vi "Send Command.vi"(6 "bytes to read":i32=256, 8 "error in (no error)":errorcluster, 9 "Get responce":bool=TRUE, 10 "Command":string="Version", 11 "RFSoC Driver in":refnum<class "RFSoC Driver.lvclass">) -> (0 "error out":errorcluster, 2 "Responce":string, 3 "RFSoC Driver out":refnum<class "RFSoC Driver.lvclass">)   [LabVIEW 2019, in "RFSoC Driver.lvclass"]
uses:
  RFSoC Driver.lvclass
  RFSoC Driver.lvclass/RFSoC Driver.ctl
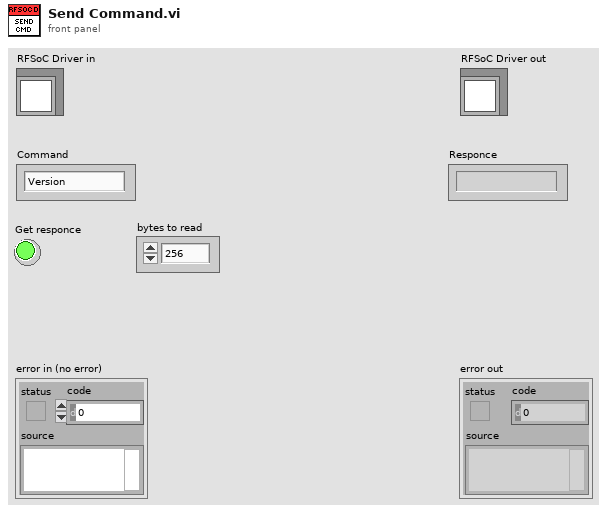
[diagram p1: front panel]
types:
  T1 = enum16{"Standard", "Buffered", "CRLF", "Immediate"}
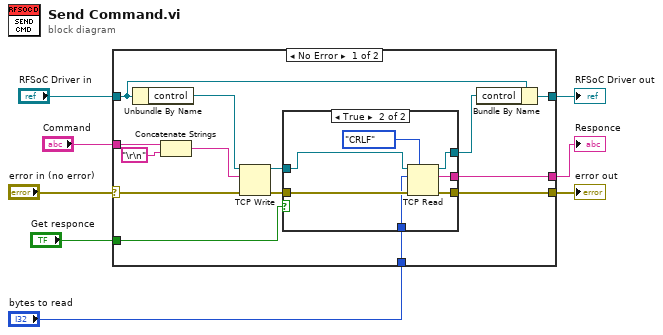
[diagram p0: block diagram]
diagram:
  n1 = case shown="No Error" "error in (no error)" {
    selector: "error in (no error)" -> [w17 w33]
    tunnel: [w14 w33] -> w7
    tunnel: [w12 w32] -> w5
    tunnel: "RFSoC Driver in" -> [w22 w32]
    tunnel: "Command" -> [w20 _]
    tunnel: "Get responce" -> [w16 _]
    tunnel: [w10 _] -> w2
    tunnel: "bytes to read" -> [w9 _]
    frame No Error {
      n2 = Unbundle By Name(w22) -> ("control"=w21:refnum<k5>)
      n3 = Concatenate Strings(w20, "\r\n") -> (w18:string)
      n4 = TCP Write(connection ID=w21, data in=w18, error in (no error)=w17) -> (connection ID out=w13:refnum<k5>, error out=w15:errorcluster)  [unwired: 1 in, 1 out]
      n5 = case shown="True" w16 {
        tunnel: w15 -> [w24 w30]
        tunnel: [w24 w29] -> w14
        tunnel: w13 -> [w23 w28]
        tunnel: [w23 w27] -> w11
        tunnel: [_ w26] -> w10
        tunnel: w9 -> [_ w25]
        frame False {
        }
        frame True {
          n6 = TCP Read(connection ID=w28, bytes to read=w25, error in (no error)=w30, 7:T1."CRLF" ("mode (standard)")) -> (connection ID out=w27:refnum<k5>, data out=w26:string, error out=w29:errorcluster)  [unwired: 1 in]
        }
      }
      n7 = Bundle By Name(cluster=w22, "control"=w11) -> (w12:refnum<class "RFSoC Driver.lvclass">)
    }
    frame Error {
    }
  }
  "error out" <- w7
  "RFSoC Driver out" <- w5
  "Responce" <- w2
